vi "9871 EPICS - FPGA - Encode Transmit FIFO U16.vi"(10 "Data Byte":u8 format="%.0x", 11 "Port# (1-4)":u8) -> (2 "U16 to Send to TX FIFO":u16 format="%016b")   [LabVIEW 2020]
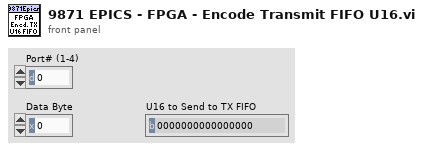
[diagram p1: front panel]
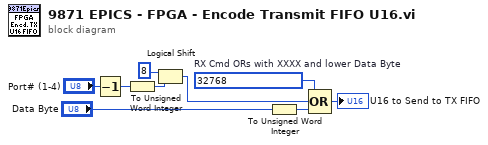
[diagram p0: block diagram]
diagram:
  w5 = u16 32768  # RX Cmd ORs with XXXX and lower Data Byte
  n1 = Decrement(x="Port# (1-4)") -> (x-1=w4:u8)
  n2 = To Unsigned Word Integer(number=w4) -> (unsigned 16bit integer=w2:u16)
  n3 = Logical Shift(y=i16 8, x=w2) -> (x << y=w1:u16)
  n4 = To Unsigned Word Integer(number="Data Byte") -> (unsigned 16bit integer=w8:u16)
  n5 = Compound Arithmetic op=OR(w5, w1, w8) -> (→"U16 to Send to TX FIFO":u16)
